vi "ZPL Query Output ON-OFF.vi"(6 "Settle (1 mS)":u32=1, 8 "error":errorcluster, 11 "VISA":refnum<visa-resource-name>) -> (0 "error out":errorcluster, 2 "Output ON":bool, 3 "VISA out":refnum<visa-resource-name>)   [LabVIEW 2015]
doc: "This VI returns a boolean:\n TRUE if the power supply output is ON and \n FALSE if the power supply output is OFF."
panel:
  # "Lambda ZPLUS \n Serial Port\n  DC Power Supplies"
  # "Read Output\nStatus"
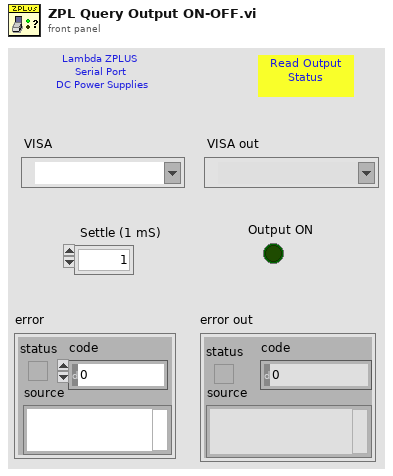
[diagram p1: front panel]
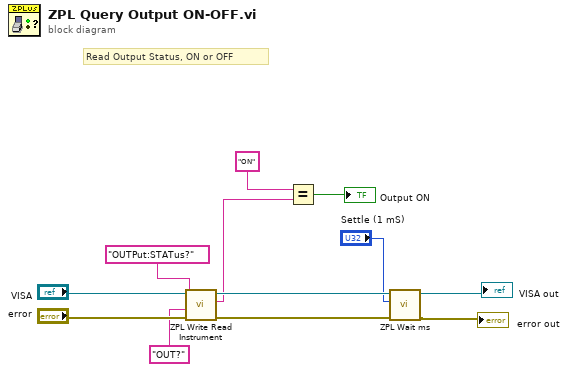
[diagram p0: block diagram]
diagram:
  # "Read Output Status, ON or OFF"
  n1 = call "ZPL Write Read Instrument.vi"("error in"="error", "Write Command/Query GEN"="OUT?" ("format string"), "Write Command/Query SCPI"="OUTPut:STATus?" ("format string"), "VISA"="VISA") -> ("error out"=w9:errorcluster, "Response"=w1:string, "VISA  out"=w10:refnum<visa-resource-name>)  [unwired: 5 in]
  n2 = Equal?(x="ON" ("format string"), y=w1) -> (x = y?=→"Output ON":bool)
  n3 = call "ZPL Wait ms.vi"("error"=w9, "Delay (1 mS)"="Settle (1 mS)", "VISA"=w10) -> ("error out"=→"error out":errorcluster, "VISA out"=→"VISA out":refnum<visa-resource-name>)  [unwired: 7 in]
